vi "Read Error.vi"(8 "error in":errorcluster, 11 "connection ID in":T1) -> (0 "error out":errorcluster, 3 "connection ID out":T1)   [LabVIEW 2010, in "NI_CCC.lvlib"]
uses:
  NI_CCC.lvlib
  <vilib>/NI/STM/TCP/TCP Connection Info.ctl
  <vilib>/NI/STM/SubVIs/MetaDataElement.ctl
  <vilib>/NI/STM/TCP/TCP Read Options.ctl
  <vilib>/NI/STM/NI STM.lvlib
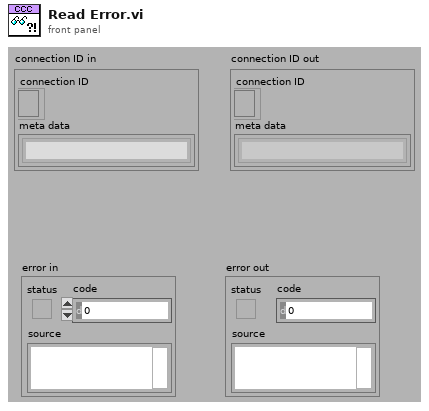
[diagram p1: front panel]
types:
  T1 = typedef "NI STM.lvlib/TCP Connection Info.ctl" = cluster{"connection ID":refnum<k5>, "meta data":T2[]}
  T2 = typedef "NI STM.lvlib/MetaDataElement.ctl" = string
  T3 = typedef "NI STM.lvlib/TCP Read Options.ctl" = cluster{"ignore timeout error":bool, "timeout ms (1000)":i32}
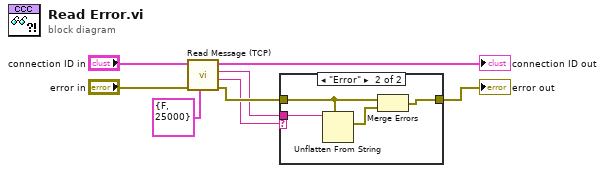
[diagram p0: block diagram]
diagram:
  n1 = call <vilib>:"Read Message (TCP).vi"("options"=T3 {"ignore timeout error"=FALSE, "timeout ms (1000)"=25000} ("Options"), "error in"="error in", "connection info in"="connection ID in") -> ("error out"=w7:errorcluster, "name"=w1:T2, "data string"=w6:string, "connection info out"=→"connection ID out":T1)  [unwired: 3 in, 2 out]
  n2 = case shown="\"Error\"" w1 {
    tunnel: w6 -> [_ w13]
    tunnel: w7 -> [w9 w12]
    tunnel: [w9 w10] -> w8
    frame Default {
      # "Unexpected Command"
    }
    frame "Error" {
      n3 = Unflatten From String(type=w12, binary string=w13) -> (value=w11:errorcluster)  [unwired: 1 in, 4 out]
      n4 = Merge Errors(w12, w11) -> (w10:errorcluster)
    }
  }
  "error out" <- w8
